vi "For ROB cluster.vi"(10 "Data in":u8[](array[numeric])) -> (1 "Type":enum16{"ROB info", "Error/Success", "Transm."}(ring)=enum."Error/Success", 2 "Data out":u8[](array[numeric]))   [LabVIEW 2016]
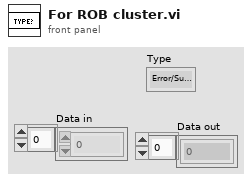
[diagram p1: front panel]
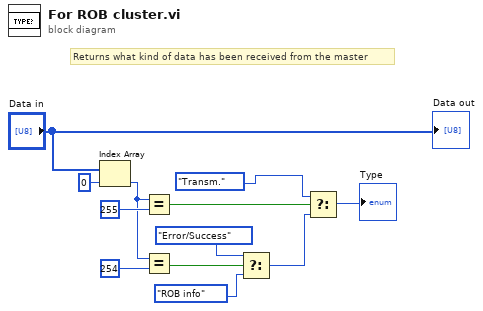
[diagram p0: block diagram]
diagram:
  # "Returns what kind of data has been received from the master"
  n1 = Index Array(array="Data in", index=0) -> (element=w8:u8)
  n2 = Equal?(x=w8, y=u8 255 ("element")) -> (x = y?=w7:bool)
  n3 = Equal?(x=w8, y=254 ("element")) -> (x = y?=w5:bool)
  n4 = Select(t=enum16{"ROB info", "Error/Success", "Transm."}."Error/Success", s=w5, f=enum16{"ROB info", "Error/Success", "Transm."}."ROB info") -> (s? t:f=w6:enum16{"ROB info", "Error/Success", "Transm."})
  n5 = Select(t=enum16{"ROB info", "Error/Success", "Transm."}."Transm.", s=w7, f=w6) -> (s? t:f=→"Type":enum16{"ROB info", "Error/Success", "Transm."})
  "Data out" <- "Data in"
